vi "Open Shutter.vi"(7 "shutter index (0)":u8, 8 "error in (no error)":errorcluster, 11 "SOL MS in":refnum<class "PL SOL Instruments MS.lvclass">) -> (0 "error out":errorcluster, 3 "SOL MS out":refnum<class "PL SOL Instruments MS.lvclass">)   [LabVIEW 2015, in "PL SOL Instruments MS.lvclass"]
doc: "Opens shutter."
uses:
  PL SOL Instruments MS.lvclass
  PL SOL Instruments MS.lvclass/PL SOL Instruments MS.ctl
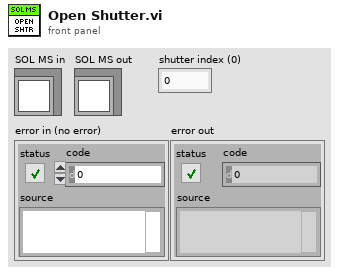
[diagram p1: front panel]
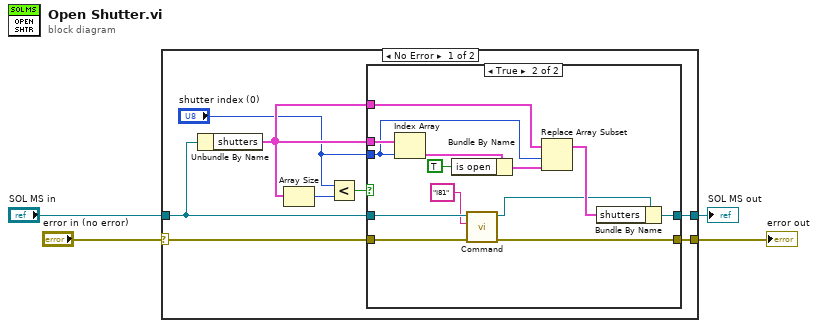
[diagram p0: block diagram]
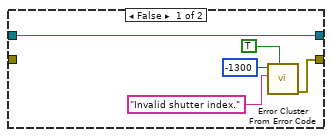
[diagram p2: hidden frame]
diagram:
  n1 = case shown="No Error" "error in (no error)" {
    selector: "error in (no error)" -> [w9 w31]
    tunnel: "SOL MS in" -> [w12 w32]
    tunnel: [w8 w32] -> w3
    tunnel: [w7 w31] -> w2
    frame No Error {
      n2 = Unbundle By Name(w12) -> ("shutters"=w6:cluster{"name":string, "is open":bool}[])
      n3 = Array Size(array=w6) -> (size(s)=w11:i32)
      n4 = Less?(x="shutter index (0)", y=w11) -> (x < y?=w10:bool)
      n5 = case shown="True" w10 {
        tunnel: w9 -> [_ w28]
        tunnel: w12 -> [w17 w29]
        tunnel: [w17 w25] -> w8
        tunnel: [w16 w24] -> w7
        tunnel: w6 -> [_ w30]
        tunnel: "shutter index (0)" -> [_ w26]
        tunnel: w6 -> [_ w27]
        frame False {
          n6 = call <vilib>:"Error Cluster From Error Code.vi"("show call chain? (False)"=TRUE, "error message (\"\")"="Invalid shutter index." ("error message (\"\")"), "error code (0)"=-1300) -> ("error out"=w16:errorcluster)  [unwired: 6 in]
        }
        frame True {
          n7 = Index Array(array=w30, index=w26) -> (element=w23:cluster{"name":string, "is open":bool})
          n8 = Bundle By Name(cluster=w23, "is open"=TRUE) -> (w22:cluster{"name":string, "is open":bool})
          n9 = call "Command.vi"("error in (no error)"=w28, "command"="I81", "SOL MS in"=w29) -> ("error out"=w24:errorcluster, "SOL MS out"=w19:refnum<class "PL SOL Instruments MS.lvclass">)  [unwired: 7 in]
          n10 = Replace Array Subset(array=w27, new element=w22, index=w26) -> (w21:cluster{"name":string, "is open":bool}[])
          n11 = Bundle By Name(cluster=w19, "shutters"=w21) -> (w25:refnum<class "PL SOL Instruments MS.lvclass">)
        }
      }
    }
    frame Error {
    }
  }
  "SOL MS out" <- w3
  "error out" <- w2
